vi "PH_SHS_Analysis_Statistician.ProcEvents.vi"(0 "i ref in":refnum<vi>, 5 "error in (no error)":errorcluster) -> (14 "i ref out":refnum<vi>, 19 "error out":errorcluster)   [LabVIEW 2014, in "PH_SHS_Analysis_Statistician.lvlib"]
doc: "This method is used to define the events the object will listen to. Add your own events here."
uses:
  PH_SHS_Analysis_Statistician.lvlib
  CSCore/BaseProcess/BaseProcess.event definition.ctl
  CSCore/CAEObj/CAEObj.event definition.ctl
  CSCore/BaseProcess/BaseProcess.descriptor string definition.ctl
  CSCore/BaseProcess/BaseProcess.lvlib
  CSCore/CAEObj/CAEObj.lvlib
  PH_Common/PH_Common.lvlib
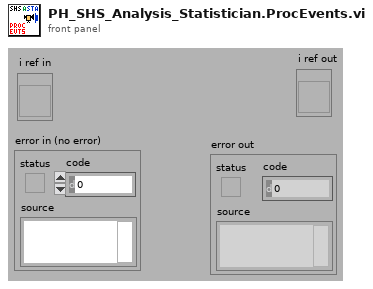
[diagram p1: front panel]
types:
  T1 = typedef "BaseProcess.lvlib/BaseProcess.event definition.ctl" = cluster{"CAEEvtDef":T2, "Data Descriptor":T3}
  T2 = typedef "CAEObj.lvlib/CAEObj.event definition.ctl" = cluster{"URL":string, "enable":bool, "ignoreResID":bool}
  T3 = typedef "BaseProcess.lvlib/BaseProcess.descriptor string definition.ctl" = string
  T4 = typedef "PH_SHS_Analysis_Statistician.lvlib/PH_SHS_Analysis_Statistician.i attribute.ctl" = cluster{"GUI Refs ":cluster{"Status":refnum<vi>, "Result Graph":refnum<vi>, "Mean Data 1":refnum<vi>, "Std Dev Data 1":refnum<vi>, "Mean Data 2":refnum<vi>, "Std Dev Data 2":refnum<vi>, "Mean Data 3":refnum<vi>, "Std Dev Data 3":refnum<vi>, "Dummy Mean":refnum<vi>, "Dummy Std Dev":refnum<vi>, "Export Data":refnum<vi>, "Data 1":refnum<vi>, "Data 2":refnum<vi>, "Data 3":refnum<vi>, "Stat or Trend":refnum<vi>, "Delete":refnum<vi>, "Analyzer":refnum<vi>, "Current Zernike Coefficients":refnum<vi>, "PtV [Lambda]":refnum<vi>, "sample length":refnum<vi>}, "Analyzer":string, "Stat or Trend":bool, "Data 1":i16, "Data 2":i16, "Data 3":i16, "Data":T5[], "sample length":i32, "Datasets strored":i32, "Dataarray Size":i32}
  T5 = typedef "PH_SHS_Analysis.lvlib/PH_SHS_Analysis.Zernike Dataset.ctl" = cluster{"State":T6, "Time Stamp":timestamp, "PtV [lambda]":dbl, "Zernicke Coefficients":T7}
  T6 = typedef "PH_StatusHandler.lvlib/PH_StatusHandler.Status.ctl" = i16
  T7 = typedef "PH_SHS_Analysis.lvlib/PH_SHS_Analysis.Zernike Coefficients.ctl" = cluster{"Tilt x":dbl, "Tilt y":dbl, "Defocus":dbl, "Astig 0°":dbl, "Astig 45°":dbl, "Coma x":dbl, "Coma y":dbl, "Spherical":dbl, "Trefoil 0°":dbl, "Trefoil 30°":dbl, "2nd Astig 0°":dbl, "2nd Astig 45°":dbl, "2nd Coma x":dbl, "2nd Coma y":dbl, "2nd Spherical":dbl}
  T8 = typedef "PH_Common.lvlib/PH_DIM.Event Declarer.ctl" = cluster{"Service Name":string, "Selector":string}
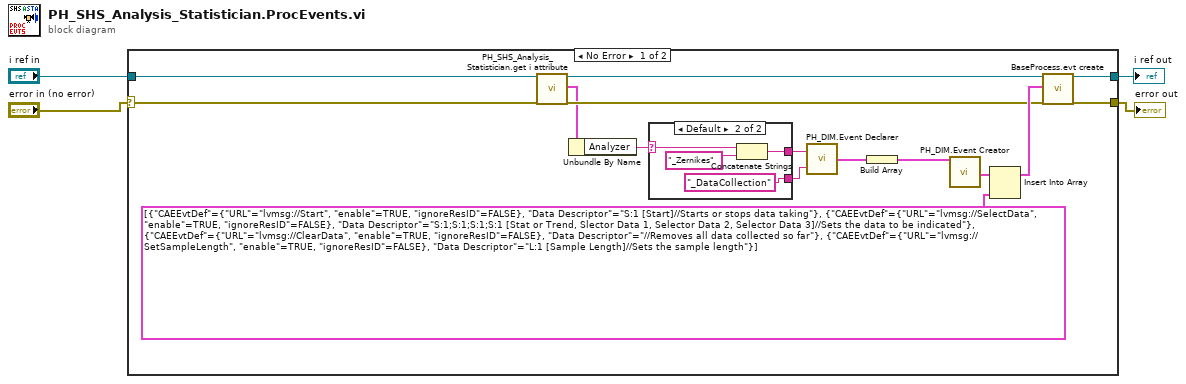
[diagram p0: block diagram]
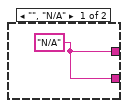
[diagram p2: hidden frame]
diagram:
  n1 = case shown="No Error" "error in (no error)" {
    selector: "error in (no error)" -> [w13 w26]
    tunnel: "i ref in" -> [w11 w25]
    tunnel: [w19 w25] -> w3
    tunnel: [w18 w26] -> w2
    frame No Error {
      n2 = call "PH_SHS_Analysis_Statistician.get i attribute.vi"("i ref in"=w11, "error in (no error)"=w13) -> ("i ref out"=w10:refnum<vi>, "i attribute"=w9:T4, "error out"=w12:errorcluster)  [unwired: 15 in]
      n3 = Unbundle By Name(w9) -> ("Analyzer"=w8:string)
      n4 = case shown="Default" w8 {
        selector: w8 -> [_ w23]
        tunnel: [w20 w22] -> w7
        tunnel: [w20 "_DataCollection"] -> w6
        frame "", "N/A" {
          w20 = "N/A"
        }
        frame Default {
          n5 = Concatenate Strings(w23, "_Zernikes") -> (w22:string)
        }
      }
      n6 = call "PH_DIM.Event Declarer.vi"("Selector"=w6, "Service Name"=w7) -> ("declared DIM Event"=w16:T8)
      n7 = Build Array(w16) -> (w5:T8[])
      n8 = call "PH_DIM.Event Creator.vi"("Trendnotifier Services"=w5) -> ("DIM Service Events"=w17:T1[])  [unwired: 18 in]
      n9 = Insert Into Array(array=w17, new element=T1[] [{"CAEEvtDef"={"URL"="lvmsg://Start", "enable"=TRUE, "ignoreResID"=FALSE}, "Data Descriptor"="S:1 [Start]//Starts or stops data taking"}, {"CAEEvtDef"={"URL"="lvmsg://SelectData", "enable"=TRUE, "ignoreResID"=FALSE}, "Data Descriptor"="S:1;S:1;S:1;S:1 [Stat or Trend, Slector Data 1, Selector Data 2, Selector Data 3]//Sets the data to be indicated"}, {"CAEEvtDef"={"URL"="lvmsg://ClearData", "enable"=TRUE, "ignoreResID"=FALSE}, "Data Descriptor"="//Removes all data collected so far"}, {"CAEEvtDef"={"URL"="lvmsg://SetSampleLength", "enable"=TRUE, "ignoreResID"=FALSE}, "Data Descriptor"="L:1 [Sample Length]//Sets the sample length"}] ("new events")) -> (w15:T1[])  [unwired: 1 in]
      n10 = call "BaseProcess.evt create.vi"("i ref in"=w10, "newEvents"=w15, "error in (no error)"=w12) -> ("i ref out"=w19:refnum<vi>, "error out"=w18:errorcluster)  [unwired: 13 in, 2 out]
    }
    frame Error {
    }
  }
  "i ref out" <- w3
  "error out" <- w2
